vi "Sine LUT 00.vi"(1 "x":sgl) -> (0 "sin(x)":sgl format="%#_8g")   [LabVIEW 2015]
uses:
  Multiply 00.vi
  Subtract 00.vi
  <vilib>/rvi/DataTransferAndStorage/Container/Common/niFpgaContainerGetUniqueNameForEmu.vi
  <vilib>/rvi/DataTransferAndStorage/Container/Common/niFpgaContainerSetEmuInfo.vi
  <vilib>/rvi/eio/common/nirviEmuReportErrorAndStop.vi
  <vilib>/rvi/DataTransferAndStorage/Container/Common/niFpgaContainerExecOnDevCompGetState.vi
  <vilib>/rvi/Emulation/niFpgaEmulationIsFPGAContextNoSignature.vi
  <vilib>/rvi/Emulation/niFpgaProcessEmulError.vi
  <vilib>/rvi/Emulation/niFpgaSctlEmulationGetInTimedLoop.vi
  <vilib>/rvi/errors/nirviReportUnexpectedCaseInternalError (U32).vi
  <vilib>/rvi/Memory/Memory_Emulation/niFpgaMemoryEmulationCacheClearOnFirstRun.vi
  <vilib>/rvi/Memory/Memory_Emulation/nirvimemoryEmulationManagerCache_MakeExclusive.vi
  <vilib>/rvi/Memory/Memory_Emulation/niFpgaMemoryEmulationValidateCache.vi
  <vilib>/rvi/Memory/Memory_Emulation/nirvimemoryEmulationManagerCache_InsertValue.vi
  <vilib>/Utility/error.llb/Clear Errors.vi
  <vilib>/rvi/Memory/Memory_Emulation/nirvimemoryEmulationManagerCache_ReleaseExclusive.vi
  <vilib>/rvi/Memory/Memory_Emulation/nirvimemoryEmulationManagerCache_GetValue.vi
  <vilib>/rvi/Memory/Memory_Emulation/nirvimemoryEmulationManagerCache_SetValue.vi
  <vilib>/rvi/Emulation/niFpgaSctlEmulationResourceMgr.vi
  Add 00.vi
  <vilib>/rvi/LocalResourceManager/LocalResourceManager.xnode
  <vilib>/rvi/DataTransferAndStorage/Container/XNode/niFpgaContainer.xnode
  <vilib>/rvi/Memory/Memory_Emulation/niFpgaMemoryEmulationRefIn.vi
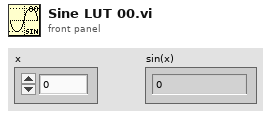
[diagram p1: front panel]
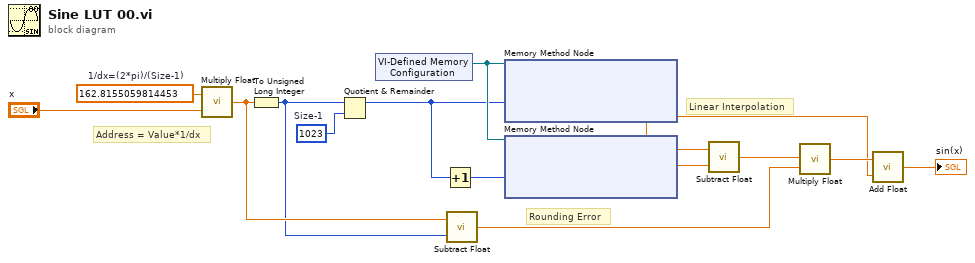
[diagram p0: block diagram]
diagram:
  w5 = u32 1023  # Size-1
  w13 = sgl 162.8155  # 1/dx=(2*pi)/(Size-1)
  # "Rounding Error"
  # "Address = Value*1/dx"
  # "Linear Interpolation"
  n1 = call-poly "Multiply Float.vi"("y"="x", "x"=w13) -> ("x*y"=w4:sgl)
  n2 = To Unsigned Long Integer(number=w4) -> (unsigned 32bit integer=w3:u32)
  n3 = Quotient & Remainder(x=w3, y=w5) -> (x-y*floor(x/y)=w6:u32)  [unwired: 1 out]
  n4 = xnode ("VI-Defined Memory Configuration")() -> ("Memory Out"=w7:refnum<k21>)
  n5 = Increment(x=w6) -> (x+1=w12:u32)
  n6 = call-poly "Subtract Float.vi"("y"=w3, "x"=w4) -> ("x*y"=w10:sgl)
  n7 = xnode ("Memory Method Node")("Address"=w6, "Memory In"=w7) -> ("Data"=w2:sgl)  [unwired: 1 out]
  n8 = xnode ("Memory Method Node")("Address"=w12, "Memory In"=w7) -> ("Data"=w8:sgl)  [unwired: 1 out]
  n9 = call-poly "Subtract Float.vi"("y"=w2, "x"=w8) -> ("x*y"=w11:sgl)
  n10 = call-poly "Multiply Float.vi"("y"=w10, "x"=w11) -> ("x*y"=w9:sgl)
  n11 = call-poly "Add Float.vi"("y"=w2, "x"=w9) -> ("x+y"=→"sin(x)":sgl)
